vi "Client.vi"() -> ()   [LabVIEW 2019]
panel:
  out "Current Data":dbl[](array[numeric])
  in  "Stop 2":bool
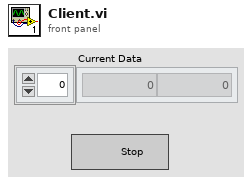
[diagram p1: front panel]
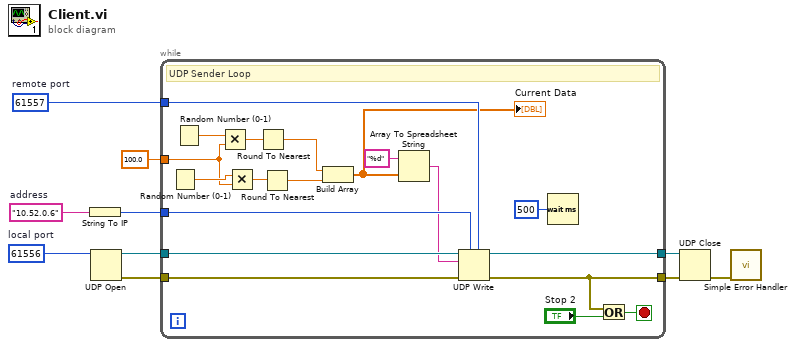
[diagram p0: block diagram]
diagram:
  w2 = u16 61557  # remote port
  w3 = u16 61556  # local port
  w8 = "10.52.0.6"  # address
  n1 = String To IP(1:w8) -> (0:w6:u32)
  n2 = UDP Open(11:w3) -> (port=w5:refnum<k16>, 0:w4:errorcluster)  [unwired: 4 in, 1 out]
  n3 = while {
    tunnel: [w24] -> w9
    tunnel: w5 -> [w29]
    tunnel: w4 -> [w28]
    tunnel: [w25] -> w10
    tunnel: w6 -> [w23]
    tunnel: w2 -> [w20]
    tunnel: 100.0 -> [w15]
    stop <- w27 stop-if-true
    # "UDP Sender Loop"
    n4 = Random Number (0-1)() -> (number: 0 to 1=w16:dbl)
    n5 = Random Number (0-1)() -> (number: 0 to 1=w17:dbl)
    n6 = Multiply(x=w17, y=w15) -> (x*y=w14:dbl)
    n7 = Multiply(x=w16, y=w15) -> (x*y=w13:dbl)
    n8 = Round To Nearest(number=w14) -> (nearest integer value=w12:dbl)
    n9 = Round To Nearest(number=w13) -> (nearest integer value=w11:dbl)
    n10 = Build Array(w12, w11) -> (w19:dbl[])
    "Current Data" <- w19
    n11 = Array To Spreadsheet String(array=w19, 3:"%d" ("format string")) -> (spreadsheet string=w21:string)  [unwired: 1 in]
    n12 = UDP Write(address=w23, port or service name=w20, connection ID=w29, data in=w21, 8:w28) -> (error out=w24:errorcluster, 3:w25:refnum<k16>)  [unwired: 1 in]
    n13 = Wait (ms)(milliseconds to wait=u32 500) -> ()  [unwired: 1 out]
    n14 = Or(x=w24, y="Stop 2") -> (x .or. y?=w27:bool)
  }
  n15 = UDP Close(connection ID=w10, 8:w9) -> (error out=w7:errorcluster)  [unwired: 1 out]
  n16 = call <vilib>:"Simple Error Handler.vi"("error in (no error)"=w7) -> ()  [unwired: 4 in, 5 out]
